vi "matrix_inversion_SGL.vi"(2 "n":i32, 3 "A":sgl[](array[numeric])) -> (0 "divide by zero detected":bool, 1 "inv(A)":sgl[](array[numeric]))   [LabVIEW 2020]
panel:
  in  "A_type":sgl format="%#_13g"
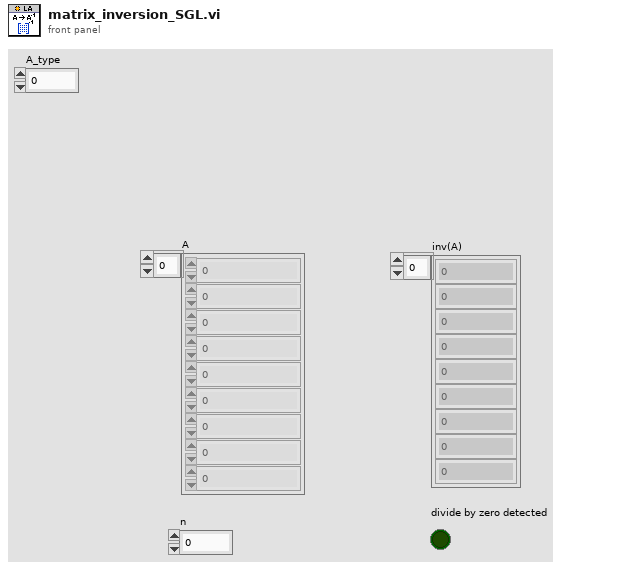
[diagram p1: front panel]
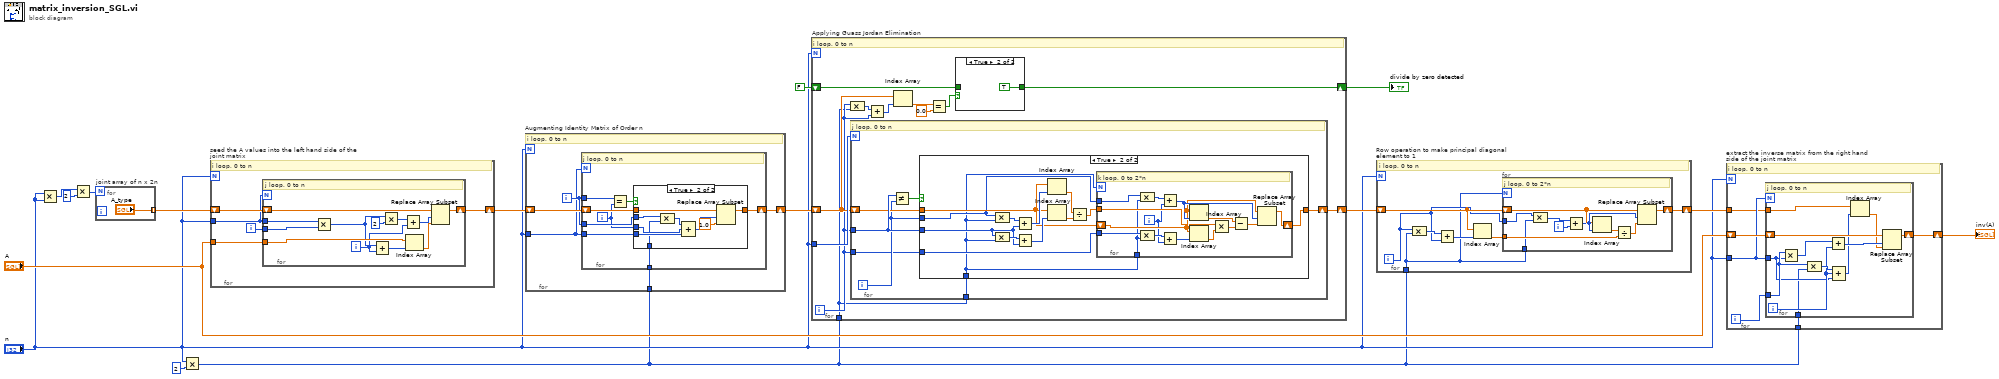
[diagram p0: block diagram]
diagram:
  n1 = Multiply(x="n", y="n") -> (x*y=w2:i32)
  n2 = Multiply(x=w2, y=2) -> (x*y=w5:i32)
  n3 = for "joint array of n x 2n" {
    N: w5 -> [_]
    tunnel: ["A_type"] -> w6 mode=indexing
  }
  n4 = Multiply(x="n", y=2) -> (x*y=w1:i32)
  n5 = for "seed the A values into the left hand side of the joint matrix" {
    N: "n" -> [_]
    shift-right: [w20] -> w7
    shift-left: w6 -> [w21]
    tunnel: "n" -> [w19]
    tunnel: "A" -> [w18]
    i -> [w17]
    # "i loop, 0 to n"
    n6 = for {
      N: w19 -> [_]
      shift-right: [w32] -> w20
      shift-left: w21 -> [w33]
      tunnel: w19 -> [w29]
      tunnel: w18 -> [w31]
      tunnel: w17 -> [w30]
      i -> [w23]
      # "j loop, 0 to n"
      n7 = Multiply(x=w29, y=w30) -> (x*y=w25:i32)
      n8 = Add(x=w25, y=w23) -> (x+y=w28:i32)
      n9 = Multiply(x=w25, y=2) -> (x*y=w24:i32)
      n10 = Add(x=w24, y=w23) -> (x+y=w22:i32)
      n11 = Index Array(array=w31, index=w28) -> (element=w27:sgl)
      n12 = Replace Array Subset(array=w33, new element=w27, index=w22) -> (w32:sgl[])
    }
  }
  n13 = for "Augmenting Identity Matrix of Order n" {
    N: "n" -> [_]
    shift-right: [w37] -> w10
    shift-left: w7 -> [w38]
    tunnel: "n" -> [w35]
    tunnel: w1 -> [w34]
    i -> [w36]
    # "i loop, 0 to n"
    n14 = for {
      N: w35 -> [_]
      tunnel: w36 -> [w46]
      shift-right: [w43] -> w37
      shift-left: w38 -> [w44]
      tunnel: w36 -> [w42]
      tunnel: w35 -> [w41]
      tunnel: w34 -> [w39]
      i -> [w40]
      # "j loop, 0 to n"
      n15 = Equal?(x=w46, y=w40) -> (x = y?=w45:bool)
      n16 = case shown="True" w45 {
        tunnel: w44 -> [w47 w56]
        tunnel: [w47 w53] -> w43
        tunnel: w42 -> [_ w54]
        tunnel: w41 -> [_ w50]
        tunnel: w40 -> [_ w51]
        tunnel: w39 -> [_ w48]
        frame False {
        }
        frame True {
          n17 = Compound Arithmetic op=MULTIPLY(w54, w48) -> (w52:i32)
          n18 = Compound Arithmetic op=ADD(w52, w51, w50) -> (w49:i32)
          n19 = Replace Array Subset(array=w56, new element=sgl 1.0 ("new element/subarray"), index=w49) -> (w53:sgl[])
        }
      }
    }
  }
  n20 = for "Applying Guass Jordan Elimination" {
    N: "n" -> [_]
    shift-right: [w62] -> w9
    shift-left: FALSE -> [w63]
    tunnel: "n" -> [w61]
    shift-right: [w58] -> w11
    shift-left: w10 -> [w60]
    tunnel: w1 -> [w57]
    i -> [w59]
    # "i loop, 0 to n"
    n21 = Compound Arithmetic op=MULTIPLY(w59, w57) -> (w67:i32)
    n22 = for {
      N: w61 -> [_]
      tunnel: w59 -> [w75]
      tunnel: w59 -> [w71]
      shift-right: [w70] -> w58
      shift-left: w60 -> [w74]
      tunnel: w57 -> [w69]
      i -> [w72]
      # "j loop, 0 to n"
      n23 = Not Equal?(x=w75, y=w72) -> (x != y?=w73:bool)
      n24 = case shown="True" w73 {
        tunnel: w75 -> [_ w83]
        tunnel: w74 -> [w76 w82]
        tunnel: w72 -> [_ w81]
        tunnel: w71 -> [_ w79]
        tunnel: [w76 w78] -> w70
        tunnel: w69 -> [_ w77]
        frame False {
        }
        frame True {
          n25 = Compound Arithmetic op=MULTIPLY(w81, w77) -> (w89:i32)
          n26 = Compound Arithmetic op=MULTIPLY(w83, w77) -> (w85:i32)
          n27 = Add(x=w89, y=w83) -> (x+y=w88:i32)
          n28 = Add(x=w85, y=w83) -> (x+y=w84:i32)
          n29 = Index Array(array=w82, index=w88) -> (element=w87:sgl)
          n30 = Index Array(array=w82, index=w84) -> (element=w86:sgl)
          n31 = Divide(x=w87, y=w86) -> (x/y=w80:sgl)
          n32 = for {
            N: w77 -> [_]
            tunnel: w81 -> [w103]
            tunnel: w80 -> [w99]
            tunnel: w79 -> [w96]
            shift-right: [w91] -> w78
            shift-left: w82 -> [w101]
            tunnel: w77 -> [w90]
            i -> [w97]
            # "k loop, 0 to 2*n"
            n33 = Compound Arithmetic op=MULTIPLY(w103, w90) -> (w104:i32)
            n34 = Compound Arithmetic op=MULTIPLY(w96, w90) -> (w98:i32)
            n35 = Add(x=w104, y=w97) -> (x+y=w102:i32)
            n36 = Add(x=w98, y=w97) -> (x+y=w95:i32)
            n37 = Index Array(array=w101, index=w102) -> (element=w93:sgl)
            n38 = Index Array(array=w101, index=w95) -> (element=w100:sgl)
            n39 = Multiply(x=w99, y=w100) -> (x*y=w94:sgl)
            n40 = Subtract(x=w93, y=w94) -> (x-y=w92:sgl)
            n41 = Replace Array Subset(array=w101, new element=w92, index=w102) -> (w91:sgl[])
          }
        }
      }
    }
    n42 = Add(x=w67, y=w59) -> (x+y=w66:i32)
    n43 = Index Array(array=w60, index=w66) -> (element=w65:sgl)
    n44 = Equal?(x=w65, y=sgl 0.0) -> (x = y?=w64:bool)
    n45 = case shown="True" w64 {
      tunnel: w63 -> [w105 _]
      tunnel: [w105 TRUE] -> w62
      frame False {
      }
      frame True {
      }
    }
  }
  "divide by zero detected" <- w9
  n46 = for "Row operation to make principal diagonal element to 1" {
    N: "n" -> [_]
    shift-right: [w108] -> w14
    shift-left: w11 -> [w111]
    tunnel: w1 -> [w107]
    i -> [w110]
    # "i loop, 0 to n"
    n47 = Compound Arithmetic op=MULTIPLY(w110, w107) -> (w113:i32)
    n48 = Add(x=w113, y=w110) -> (x+y=w112:i32)
    n49 = Index Array(array=w111, index=w112) -> (element=w109:sgl)
    n50 = for {
      N: w107 -> [_]
      tunnel: w110 -> [w123]
      tunnel: w109 -> [w119]
      shift-right: [w117] -> w108
      shift-left: w111 -> [w118]
      tunnel: w107 -> [w114]
      i -> [w121]
      # "j loop, 0 to 2*n"
      n51 = Compound Arithmetic op=MULTIPLY(w123, w114) -> (w122:i32)
      n52 = Add(x=w122, y=w121) -> (x+y=w116:i32)
      n53 = Index Array(array=w118, index=w116) -> (element=w120:sgl)
      n54 = Divide(x=w120, y=w119) -> (x/y=w115:sgl)
      n55 = Replace Array Subset(array=w118, new element=w115, index=w116) -> (w117:sgl[])
    }
  }
  n56 = for "extract the inverse matrix from the right hand side of the joint matrix" {
    N: "n" -> [_]
    tunnel: "n" -> [w126]
    shift-right: [w128] -> w13
    shift-left: "A" -> [w129]
    tunnel: w14 -> [w125]
    tunnel: w1 -> [w124]
    i -> [w127]
    # "i loop, 0 to n"
    n57 = for {
      N: w126 -> [_]
      shift-right: [w140] -> w128
      shift-left: w129 -> [w141]
      tunnel: w127 -> [w137]
      tunnel: w126 -> [w134]
      tunnel: w125 -> [w132]
      tunnel: w124 -> [w130]
      i -> [w135]
      # "j loop, 0 to n"
      n58 = Multiply(x=w137, y=w134) -> (x*y=w139:i32)
      n59 = Compound Arithmetic op=MULTIPLY(w137, w130) -> (w136:i32)
      n60 = Add(x=w139, y=w135) -> (x+y=w138:i32)
      n61 = Compound Arithmetic op=ADD(w136, w135, w134) -> (w133:i32)
      n62 = Index Array(array=w132, index=w133) -> (element=w131:sgl)
      n63 = Replace Array Subset(array=w141, new element=w131, index=w138) -> (w140:sgl[])
    }
  }
  "inv(A)" <- w13
